vi "Centrifuge Close Selection.vi"(8 "error in (no error)":errorcluster, 11 "Pump Settings In":T1={"Output Device"=enum."Default", "EPOS4 Settings"={"VISA resource name"="", "Simulated?"=FALSE, "axis"={"keyHandle"=0, "nodeId"=1}}}) -> (0 "error out":errorcluster, 1 "Connection Error":bool, 3 "Pump Settings Out":T1={"Output Device"=enum."Default", "EPOS4 Settings"={"VISA resource name"="", "Simulated?"=FALSE, "axis"={"keyHandle"=0, "nodeId"=1}}})   [LabVIEW 2018, in "Centrifuge Module.lvlib" / "Centrifuge Module Engine.lvlib"]
uses:
  Measure Instrument/Centrifuge Module Engine.lvlib
  Measure Instrument/Centrifuge Settings Cluster.ctl
  EPOS4/Controls/Device Selection.ctl
  EPOS4/Controls/EPOS Communication Settings.ctl
  Centrifuge Module.lvlib
  EPOS4/EPOS4.lvlib
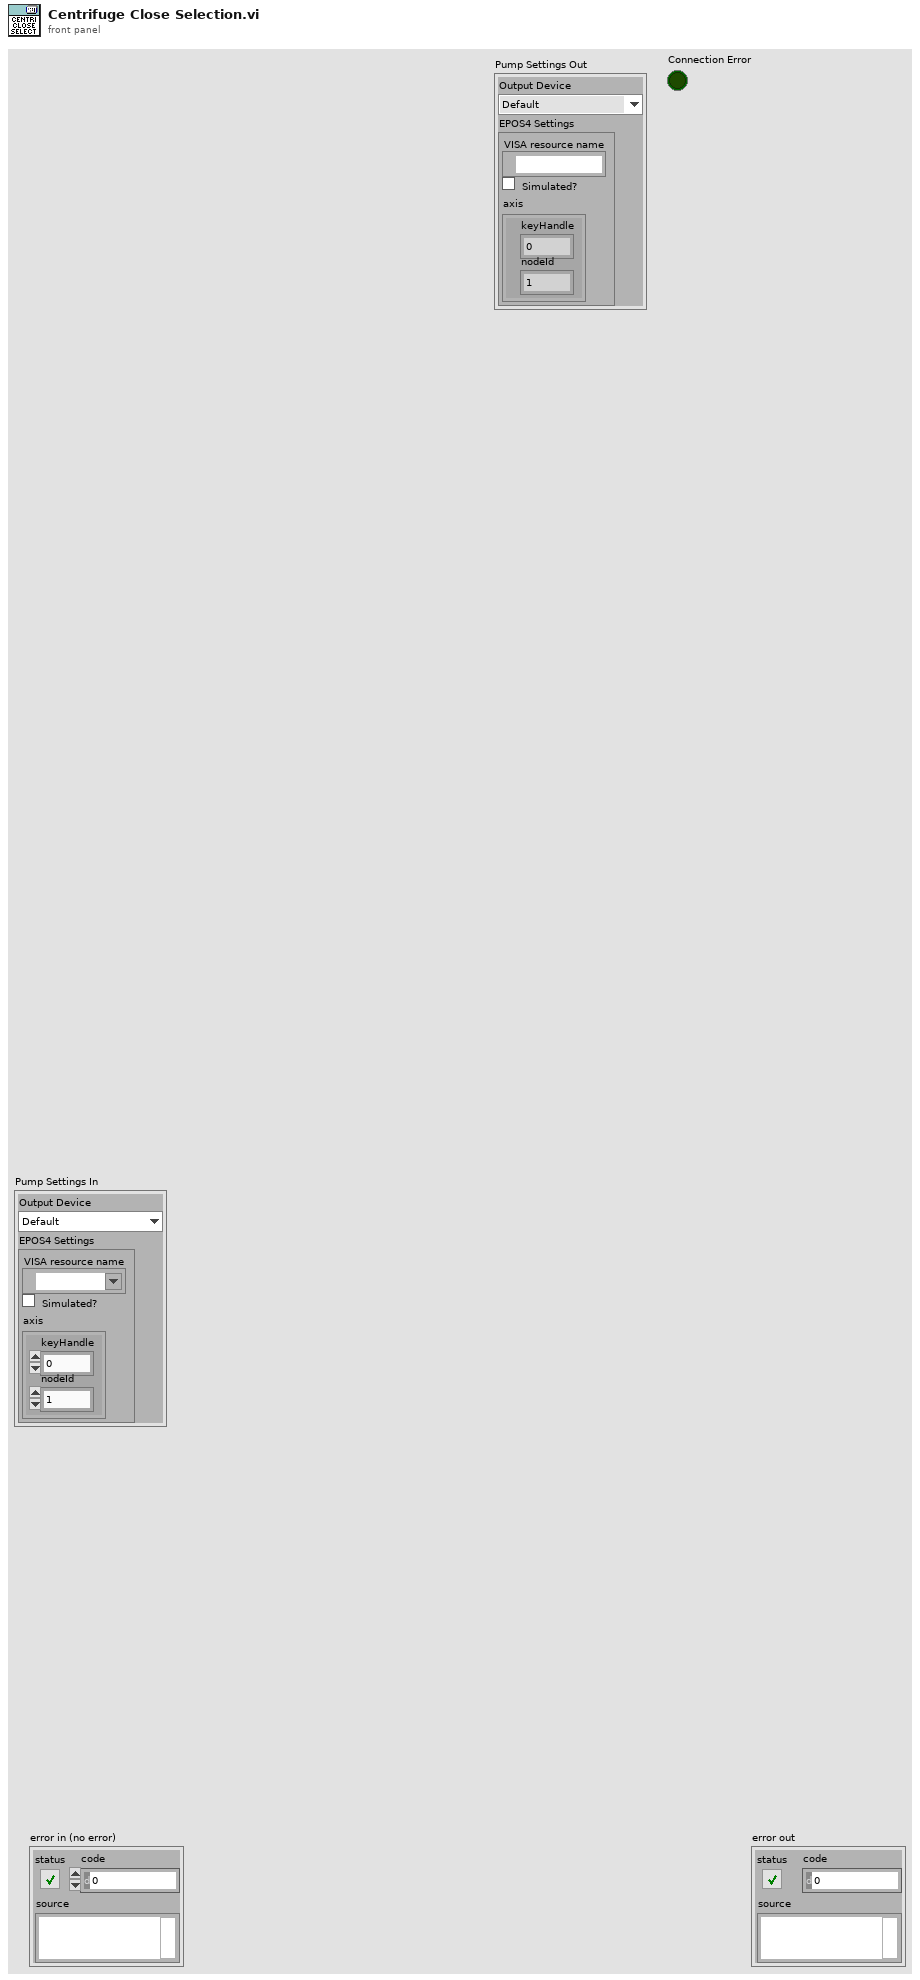
[diagram p1: front panel]
types:
  T1 = typedef "Centrifuge Module.lvlib/Centrifuge Settings Cluster.ctl" = cluster{"Output Device":T2, "EPOS4 Settings":T3}
  T2 = typedef "Device Selection.ctl" = enum16{"Default", "EPOS4"}
  T3 = typedef "EPOS4.lvlib/EPOS Communication Settings.ctl" = cluster{"VISA resource name":refnum<visa-resource-name>, "Simulated?":bool, "axis":cluster{"keyHandle":u32, "nodeId":u16}}
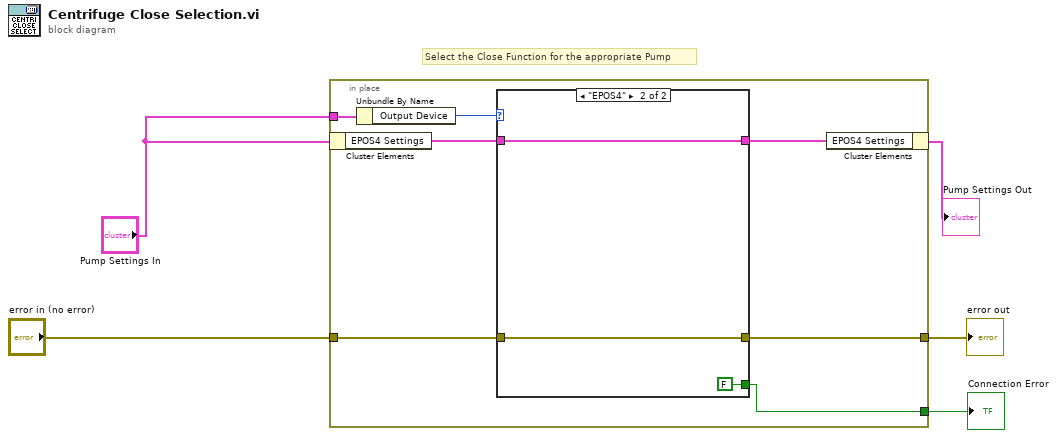
[diagram p0: block diagram]
diagram:
  # "Select the Close Function for the appropriate Pump"
  n1 = in-place {
    in-place-border: "error in (no error)" -> [w11]
    in-place-border: [w10] -> w4
    in-place-border: "Pump Settings In" -> [w9]
    in-place-border: [w8] -> w3
    n2 = in-place-cluster #1("Pump Settings In") -> ("EPOS4 Settings"=w7:T3)
    n3 = Unbundle By Name(w9) -> ("Output Device"=w12:T2)
    n4 = case shown="\"EPOS4\"" w12 {
      tunnel: w7 -> [w14 w17]
      tunnel: [w14 w17] -> w6
      tunnel: [w13 w16] -> w10
      tunnel: w11 -> [w13 w16]
      tunnel: [_ FALSE ("Connection Error")] -> w8
      frame "Default", Default {
      }
      frame "EPOS4" {
      }
    }
    n5 = in-place-cluster #1("EPOS4 Settings"=w6) -> (→"Pump Settings Out":T1)
  }
  "error out" <- w4
  "Connection Error" <- w3
